vi "LEIN Q Uniqe command.vi"(0 "LEIN custom reply Q":T1, 1 "Retry on err (F)":bool, 5 "Custom Q(F)":bool, 7 "CMD":T2, 11 "error in":errorcluster, 12 "priority(F)":bool) -> (15 "error out":errorcluster)   [LabVIEW 2011]
uses:
  Defenitions/LEIN CMD Cluster.ctl
  Defenitions/LEIN CMD List.ctl
  Defenitions/LEIN custom reply Q.ctl
  Defenitions/LEIN Reply Holder.ctl
  Defenitions/LEIN cycle holder.ctl
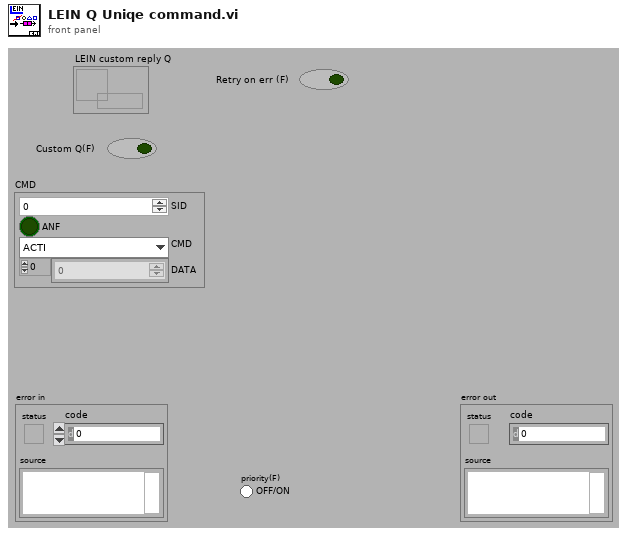
[diagram p1: front panel]
types:
  T1 = typedef "LEIN custom reply Q.ctl" = refnum<queue>
  T2 = typedef "LEIN CMD Cluster.ctl" = cluster{"SID":u8, "ANF":bool, "CMD":T3, "DATA":u8[]}
  T3 = typedef "LEIN CMD List.ctl" = enum8{"ACTI", "TASK", "RES0", "STAT", "RES1", "RES2", "RES3", "USER"}
  T4 = typedef "LEIN cycle holder.ctl" = cluster{"CMD":T2, "Retry if  unsucessful":bool, "LEIN reply holder":T5, "Reply in custom Q":bool, "LEIN custom reply Q":T1}
  T5 = typedef "LEIN Reply Holder.ctl" = cluster{"Reply msg(cmdif no reply)":T2, "Reply time":timestamp, "Valid reply":bool}
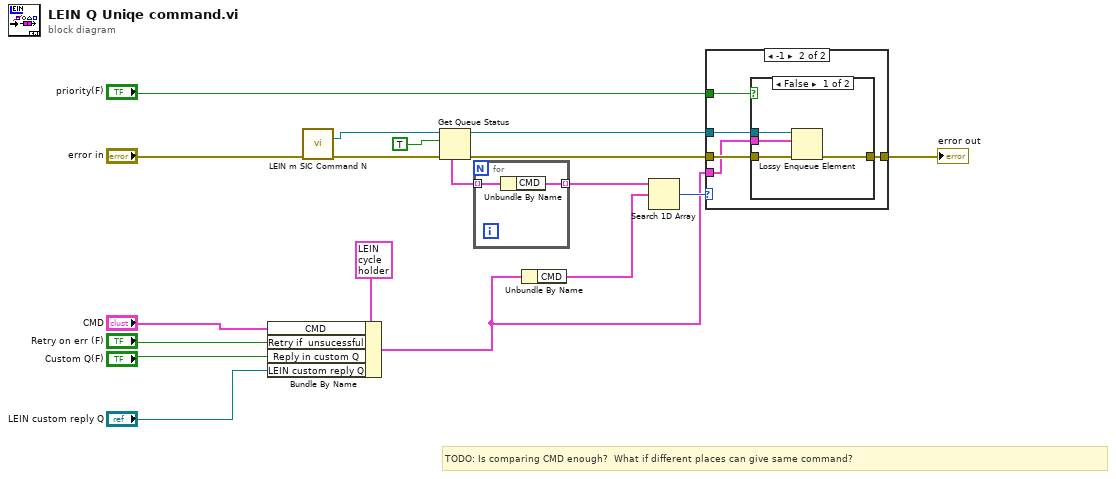
[diagram p0: block diagram]
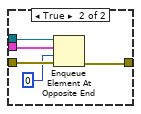
[diagram p3: hidden frame]
diagram:
  # "TODO: Is comparing CMD enough?  What if different places can give same command?"
  n1 = Bundle By Name(cluster=T4 {"CMD"={"SID"=0, "ANF"=FALSE, "CMD"=enum."ACTI", "DATA"=[]}, "Retry if  unsucessful"=FALSE, "LEIN reply holder"={"Reply msg(cmdif no reply)"={"SID"=0, "ANF"=FALSE, "CMD"=enum."ACTI", "DATA"=[]}, "Reply time"=timestamp(0 s since 1904-01-01), "Valid reply"=FALSE}, "Reply in custom Q"=FALSE, "LEIN custom reply Q"=refnum} ("element"), "CMD"="CMD", "Retry if  unsucessful"="Retry on err (F)", "Reply in custom Q"="Custom Q(F)", "LEIN custom reply Q"="LEIN custom reply Q") -> (w6:T4)
  n2 = call "LEIN m SIC Command N.vi"("error in (no error)"="error in") -> ("queue out"=w13:refnum<queue>, "error out"=w18:errorcluster)  [unwired: 13 in]
  n3 = Get Queue Status(queue=w13, return elements? (F)=TRUE, error in (no error)=w18) -> (queue out=w17:refnum<queue>, error out=w16:errorcluster, elements=w8:T4[])  [unwired: 5 out]
  n4 = for {
    tunnel: w8 -> [w20] mode=indexing
    tunnel: [w19] -> w7 mode=indexing
    n5 = Unbundle By Name(w20) -> ("CMD"=w19:T2)
  }
  n6 = Unbundle By Name(w6) -> ("CMD"=w5:T2)
  n7 = Search 1D Array(1D array=w7, element=w5) -> (index of element=w14:i32)  [unwired: 1 in]
  n8 = case shown="-1" w14 {
    tunnel: [w21 w25] -> w15
    tunnel: w16 -> [w21 w26]
    tunnel: w6 -> [_ w23]
    tunnel: w17 -> [_ w24]
    tunnel: "priority(F)" -> [_ w22]
    frame 0, Default {
    }
    frame -1 {
      n9 = case shown="False" w22 {
        tunnel: w26 -> [w30 w35]
        tunnel: [w29 w34] -> w25
        tunnel: w24 -> [w28 w32]
        tunnel: w23 -> [w27 w33]
        frame False {
          n10 = Lossy Enqueue Element(queue=w28, element=w27, error in (no error)=w30) -> (error out=w29:errorcluster)  [unwired: 3 out]
        }
        frame True {
          n11 = Enqueue Element At Opposite End(queue=w32, element=w33, timeout in ms (-1)=0, error in (no error)=w35) -> (error out=w34:errorcluster)  [unwired: 2 out]
        }
      }
    }
  }
  "error out" <- w15
